vi "Read ObjectiveBook.vi"(8 "error in (no error)":errorcluster, 11 "Evaluator in":refnum<class "Evaluator.lvclass">) -> (0 "error out":errorcluster, 2 "ObjectiveBook":refnum<class "Objective.lvclass">[](array[class]), 3 "Evaluator out":refnum<class "Evaluator.lvclass">)   [LabVIEW 2023, in "Evaluator.lvclass"]
uses:
  Evaluator.lvclass
  Objective_class/Objective.lvclass
  Evaluator.lvclass/Evaluator.ctl
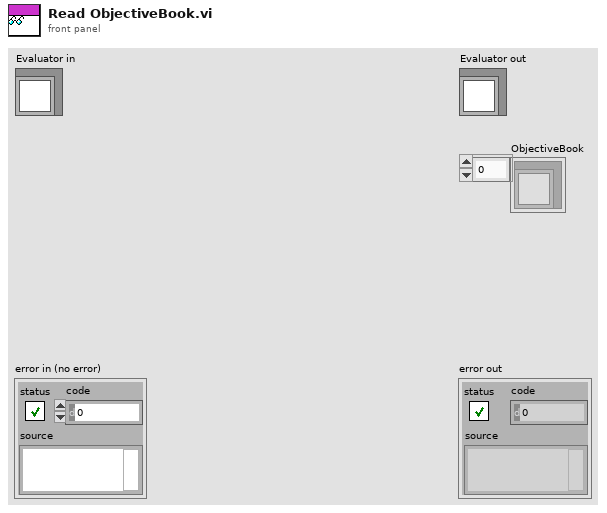
[diagram p1: front panel]
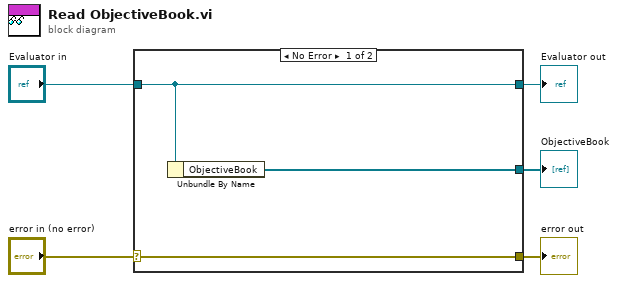
[diagram p0: block diagram]
diagram:
  n1 = case shown="No Error" "error in (no error)" {
    selector: "error in (no error)" -> [w8 w9]
    tunnel: [w8 w9] -> w4
    tunnel: [w7 w10] -> w2
    tunnel: "Evaluator in" -> [w7 w10]
    tunnel: [w6 _] -> w1
    frame No Error {
      n2 = Unbundle By Name(w7) -> ("ObjectiveBook"=w6:refnum<class "Objective.lvclass">[])
    }
    frame Error {
    }
  }
  "error out" <- w4
  "Evaluator out" <- w2
  "ObjectiveBook" <- w1
